vi "I2C Position Sensor Rotation.vi"() -> (0 "Rotation Position":i32, 3 "Elevator Rotation Sensor Working":bool)   [LabVIEW 2014]
uses:
  Robot Global Data.vi
panel:
  out "Elevator Speed  Chart":dbl(graph)
  out "Previous Time 2":u32
  out "Current Time":u32
  out "Number of Rotations":i16
  out "Elevator Rotation Sensor Position":dbl(knob) scale=0.0..1.0
  out "RotationFinal":dbl
  out "AngleRaw":u16
  out "Diag codes":u8
  out "MagnetFieldStregth":u8
  out "Rotation Sensor Data Out":u8[](array[numeric])
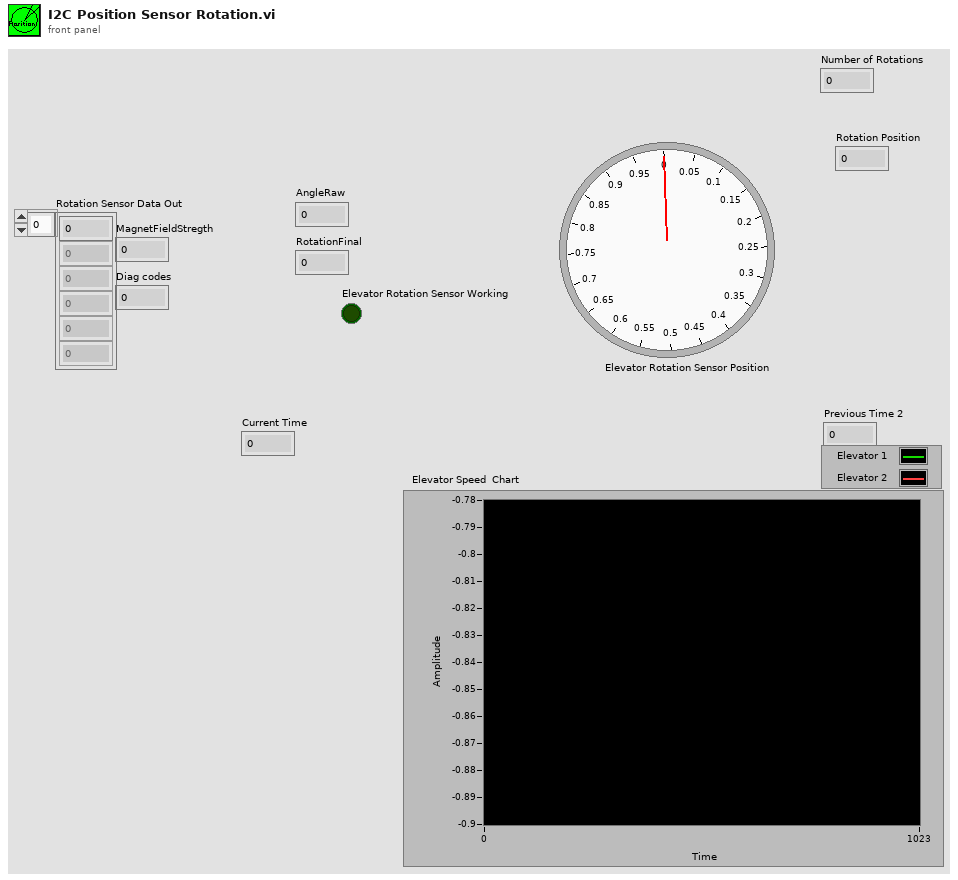
[diagram p1: front panel]
types:
  T1 = typedef "WPI_I2CDevRef.ctl" = cluster{"DevStatus":errorcluster, "Controller":T2, "Device Address":u8, "Handle":i32, "I2C Bus":T3}
  T2 = typedef "FPGA_TypedefDigitalModule.ctl" = enum16{"Controller 1"}
  T3 = typedef "i2c_bus.ctl" = enum16{"I2C On-Board", "I2C MXP", "Invalid"}
  T4 = cluster{"Boolean array[0]":bool, "Boolean array[1]":bool, "Boolean array[2]":bool, "Boolean array[3]":bool, "Boolean array[4]":bool, "Boolean array[5]":bool, "Boolean array[6]":bool, "Boolean array[7]":bool}
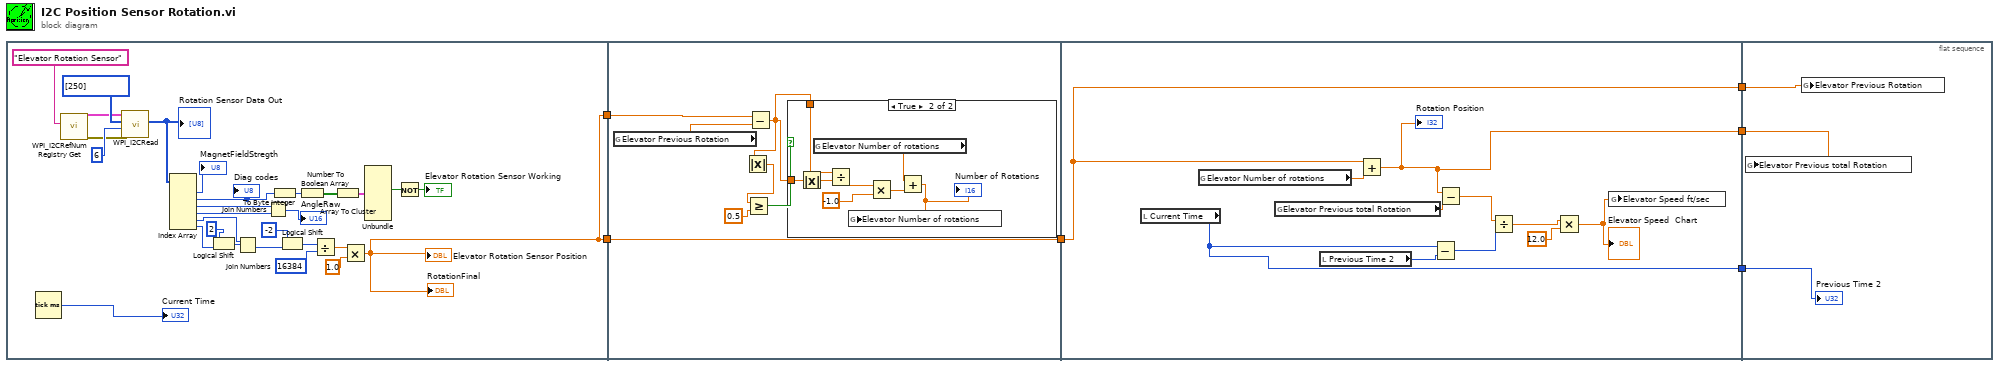
[diagram p0: block diagram]
diagram:
  n1 = flat-sequence {
    tunnel: [w8] -> w6
    tunnel: [w8] -> w5
    tunnel: w6 -> [w35]
    tunnel: w5 -> [w41]
    tunnel: [w35] -> w4
    tunnel: w4 -> [w54]
    tunnel: [w54] -> w3
    tunnel: [w53] -> w2
    tunnel: [w50] -> w1
    tunnel: w3 -> [w63]
    tunnel: w2 -> [w62]
    tunnel: w1 -> [w61]
    frame #0 {
      n2 = Tick Count (ms)() -> (millisecond timer value=→"Current Time":u32)
      n3 = call <vilib>:"WPI_I2CRefNum Registry Get.vi"("refnum name"="Elevator Rotation Sensor") -> ("error out"=w11:errorcluster, "I2CDevRef"=w9:T1)  [unwired: 9 in]
      n4 = call <vilib>:"WPI_I2CRead.vi"("error in (no error)"=w11, "I2CBytesToRead"=u8 6, "I2CRegister"=u8[] [250], "I2CDevRef"=w9) -> ("Data Out"=w14:u8[])  [unwired: 5 in, 2 out]
      "Rotation Sensor Data Out" <- w14
      n5 = Index Array(array=w14) -> (element #1=→"MagnetFieldStregth":u8, element #2=w22:u8, element #3=w17:u8, element #4=w18:u8, element #5=w19:u8, element #6=w27:u8)  [unwired: 6 in]
      "Diag codes" <- w22
      n6 = Logical Shift(y=i16 2, x=w27) -> (x << y=w28:u8)
      n7 = Join Numbers(hi=w19, lo=w28) -> ((hi.lo)=w29:u16)
      n8 = Join Numbers(hi=w17, lo=w18) -> ((hi.lo)=→"AngleRaw":u16)
      n9 = To Byte Integer(number=w22) -> (8bit integer=w21:i8)
      n10 = Logical Shift(y=i16 -2, x=w29) -> (x << y=w31:u16)
      n11 = Number To Boolean Array(number=w21) -> (Boolean array=w23:bool[])
      n12 = Divide(x=w31, y=u16 16384) -> (x/y=w33:dbl)
      n13 = Array To Cluster(array=w23) -> (cluster=w20:T4)
      n14 = Multiply(x=w33, y=1.0) -> (x*y=w8:dbl)
      "RotationFinal" <- w8
      "Elevator Rotation Sensor Position" <- w8
      n15 = Unbundle(w20) -> ("Boolean array[3]"=w24:bool)  [unwired: 7 out]
      n16 = Not(x=w24) -> (.not. x?=→"Elevator Rotation Sensor Working":bool)
    }
    frame #1 {
      n17 = global read "Robot Global Data.vi" "Elevator Previous Rotation"() -> (w39:dbl)
      n18 = Subtract(x=w41, y=w39) -> (x-y=w36:dbl)
      n19 = Absolute Value(x=w36) -> (abs(x)=w38:dbl)
      n20 = Greater Or Equal?(x=w38, y=0.5) -> (x >= y?=w37:bool)
      n21 = case shown="True" w37 {
        tunnel: w36 -> [_ w49]
        tunnel: w36 -> [_ w48]
        frame False {
        }
        frame True {
          n22 = Absolute Value(x=w48) -> (abs(x)=w47:dbl)
          n23 = global read "Robot Global Data.vi" "Elevator Number of rotations"() -> (w42:dbl)
          n24 = Divide(x=w49, y=w47) -> (x/y=w44:dbl)
          n25 = Multiply(x=w44, y=-1.0) -> (x*y=w45:dbl)
          n26 = Add(x=w42, y=w45) -> (x+y=w43:dbl)
          "Number of Rotations" <- w43
          n27 = global write "Robot Global Data.vi" "Elevator Number of rotations"(w43) -> ()
        }
      }
    }
    frame #2 {
      n28 = local read "Current Time"() -> (w53:u32)
      n29 = global read "Robot Global Data.vi" "Elevator Number of rotations"() -> (w60:dbl)
      n30 = global read "Robot Global Data.vi" "Elevator Previous total Rotation"() -> (w58:dbl)
      n31 = local read "Previous Time 2"() -> (w59:u32)
      n32 = Add(x=w54, y=w60) -> (x+y=w50:dbl)
      "Rotation Position" <- w50
      n33 = Subtract(x=w53, y=w59) -> (x-y=w57:u32)
      n34 = Subtract(x=w50, y=w58) -> (x-y=w51:dbl)
      n35 = Divide(x=w51, y=w57) -> (x/y=w52:dbl)
      n36 = Multiply(x=w52, y=12.0) -> (x*y=w55:dbl)
      "Elevator Speed  Chart" <- w55
      n37 = global write "Robot Global Data.vi" "Elevator Speed ft/sec"(w55) -> ()
    }
    frame #3 {
      n38 = global write "Robot Global Data.vi" "Elevator Previous total Rotation"(w61) -> ()
      n39 = global write "Robot Global Data.vi" "Elevator Previous Rotation"(w63) -> ()
      "Previous Time 2" <- w62
    }
  }
